vi "Get All Platforms.vi"(8 "error in (no error)":errorcluster, 11 "PlatformManager in":refnum<class "PlatformManager.lvclass">) -> (0 "error out":errorcluster, 2 "Platforms":refnum<class "Platform.lvclass">[](array[class]), 3 "PlatformManager out":refnum<class "PlatformManager.lvclass">)   [LabVIEW 2020, in "PicoG-Core.lvlib" / "PlatformManager.lvclass"]
uses:
  PlatformManager.lvclass
  Platform/Platform.lvclass
  PlatformManager.lvclass/PlatformManager.ctl
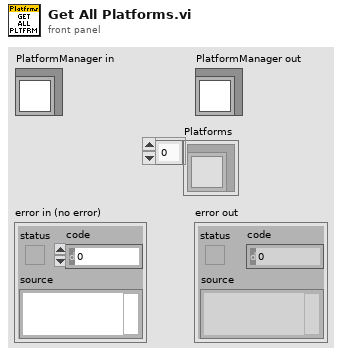
[diagram p1: front panel]
types:
  T1 = typedef "PicoG-Core.lvlib/PlatformManager.lvclass/Ref Data.ctl" = cluster{"Platforms":refnum<class "Platform.lvclass">[]}
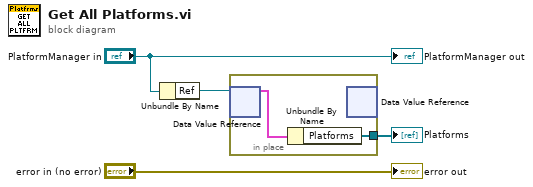
[diagram p0: block diagram]
diagram:
  n1 = Unbundle By Name("PlatformManager in") -> ("Ref"=w3:refnum<data-value>)
  n2 = in-place {
    in-place-border: [w5] -> w1
    n3 = in-place-dvr #1(w3) -> (w6:T1)  [unwired: 1 out]
    n4 = Unbundle By Name(w6) -> ("Platforms"=w5:refnum<class "Platform.lvclass">[])
    n5 = in-place-dvr #1() -> ()  [unwired: 1 in, 2 out]
  }
  "Platforms" <- w1
  "error out" <- "error in (no error)"
  "PlatformManager out" <- "PlatformManager in"
